vi "KB-产品统计.vi"(7 "file path (dialog if empty)":path=path "E:/Users/HEZHIFENG/Desktop/image Picture#2 Balck/20160927.xls", 9 "限位表格":string[][](table)=[["0.2", "0", "0.25", "0", "0.1", "0", "10", "-10", "金色"], ["0.2", "0", "0.25", "0", "0.1", "0", "10", "-10", "金色"], ["0.2", "0", "0.25", "0", "0.1", "0", "10", "-10", "金色"], ["0.2", "0", "0.25", "0", "0.1", "0", "10", "-10", "金色"], ["0.2", "0", "0.25", "0", "0.1", "0", "10", "-10", "金色"], ["0.2", "0", "0.25", "0", "0.1", "0", "10", "-10", "金色"], ["0.2", "0", "0.25", "0", "0.1", "0", "10", "-10", "银色"], ["0.2", "0", "0.25", "0", "0.1", "0", "10", "-10", "银色"], ["0.2", "0", "0.25", "0", "0.1", "0", "10", "-10", "银色"], ["0.2", "0", "0.25", "0", "0.1", "0", "10", "-10", "银色"], ["0.2", "0", "0.25", "0", "0.1", "0", "10", "-10", "金色"], ["0.2", "0", "0.25", "0", "0.1", "0", "10", "-10", "金色"], ["0.2", "0", "0.25", "0", "0.1", "0", "10", "-10", "金色"], ["0.2", "0", "0.25", "0", "0.1", "0", "10", "-10", "金色"], ["0.2", "0", "0.25", "0", "0.1", "0", "10", "-10", "金色"], ["0.2", "0", "0.25", "0", "0.1", "0", "10", "-10", "金色"], ["0.2", "0", "0.25", "0", "0.1", "0", "10", "-10", "金色"], ["0.2", "0", "0.25", "0", "0.1", "0", "10", "-10", "金色"], ["0.2", "0", "0.25", "0", "0.1", "0", "10", "-10", "金色"], ["0.2", "0", "0.25", "0", "0.1", "0", "10", "-10", "金色"], ["0.2", "0", "0.25", "0", "0.1", "0", "10", "-10", "金色"], ["0.2", "0", "0.25", "0", "0.1", "0", "10", "-10", "金色"], ["0.2", "0", "0.25", "0", "0.1", "0", "10", "-10", "金色"], ["0.2", "0", "0.25", "0", "0.1", "0", "10", "-10", "金色"], ["0.2", "0", "0.25", "0", "0.1", "0", "10", "-10", "金色"], ["0.2", "0", "0.25", "0", "0.1", "0", "10", "-10", "金色"], ["0.2", "0", "0.25", "0", "0.1", "0", "10", "-10", "金色"], ["0.2", "0", "0.25", "0", "0.1", "0", "10", "-10", "金色"], ["0.2", "0", "0.25", "0", "0.1", "0", "10", "-10", "金色"], ["0.2", "0", "0.25", "0", "0.1", "0", "10", "-10", "金色"], ["0.2", "0", "0.25", "0", "0.1", "0", "10", "-10", "金色"]], 10 "结束时间":string(combo)="24", 11 "起始时间":string(combo)="01") -> (1 "Tab同心度":string[][](table)=[["0", "0", "0", "0", "0"]], 2 "Tab高度差":string[][](table)=[["165", "20", "1", "0", "0"]], 3 "Tab":string[][](table)=[["1", "", "255", "N/A", "N/A", "N/A", "465"], ["2", "", "N/A", "250", "N/A", "N/A", "N/A"], ["3", "", "N/A", "N/A", "20", "N/A", "N/A"], ["4", "", "N/A", "N/A", "N/A", "10", "N/A"]])   [LabVIEW 2015]
uses:
  <vilib>/Utility/miscctls.llb/LVRowAndColumnTypeDef.ctl
  <vilib>/Utility/file.llb/Read Delimited Spreadsheet (string).vi
panel:
  out "数组":string[](array[string])
  out "子数组":string[](array[string])
  out "已删除元素的数组子集":string[][](array[string])
  out "输出簇":T1
  out "OK 个数":string
  out "混装 个数":string
  out "同心度NG 个数":string
  out "高度差NG 个数":string
  out "漏料个数":string
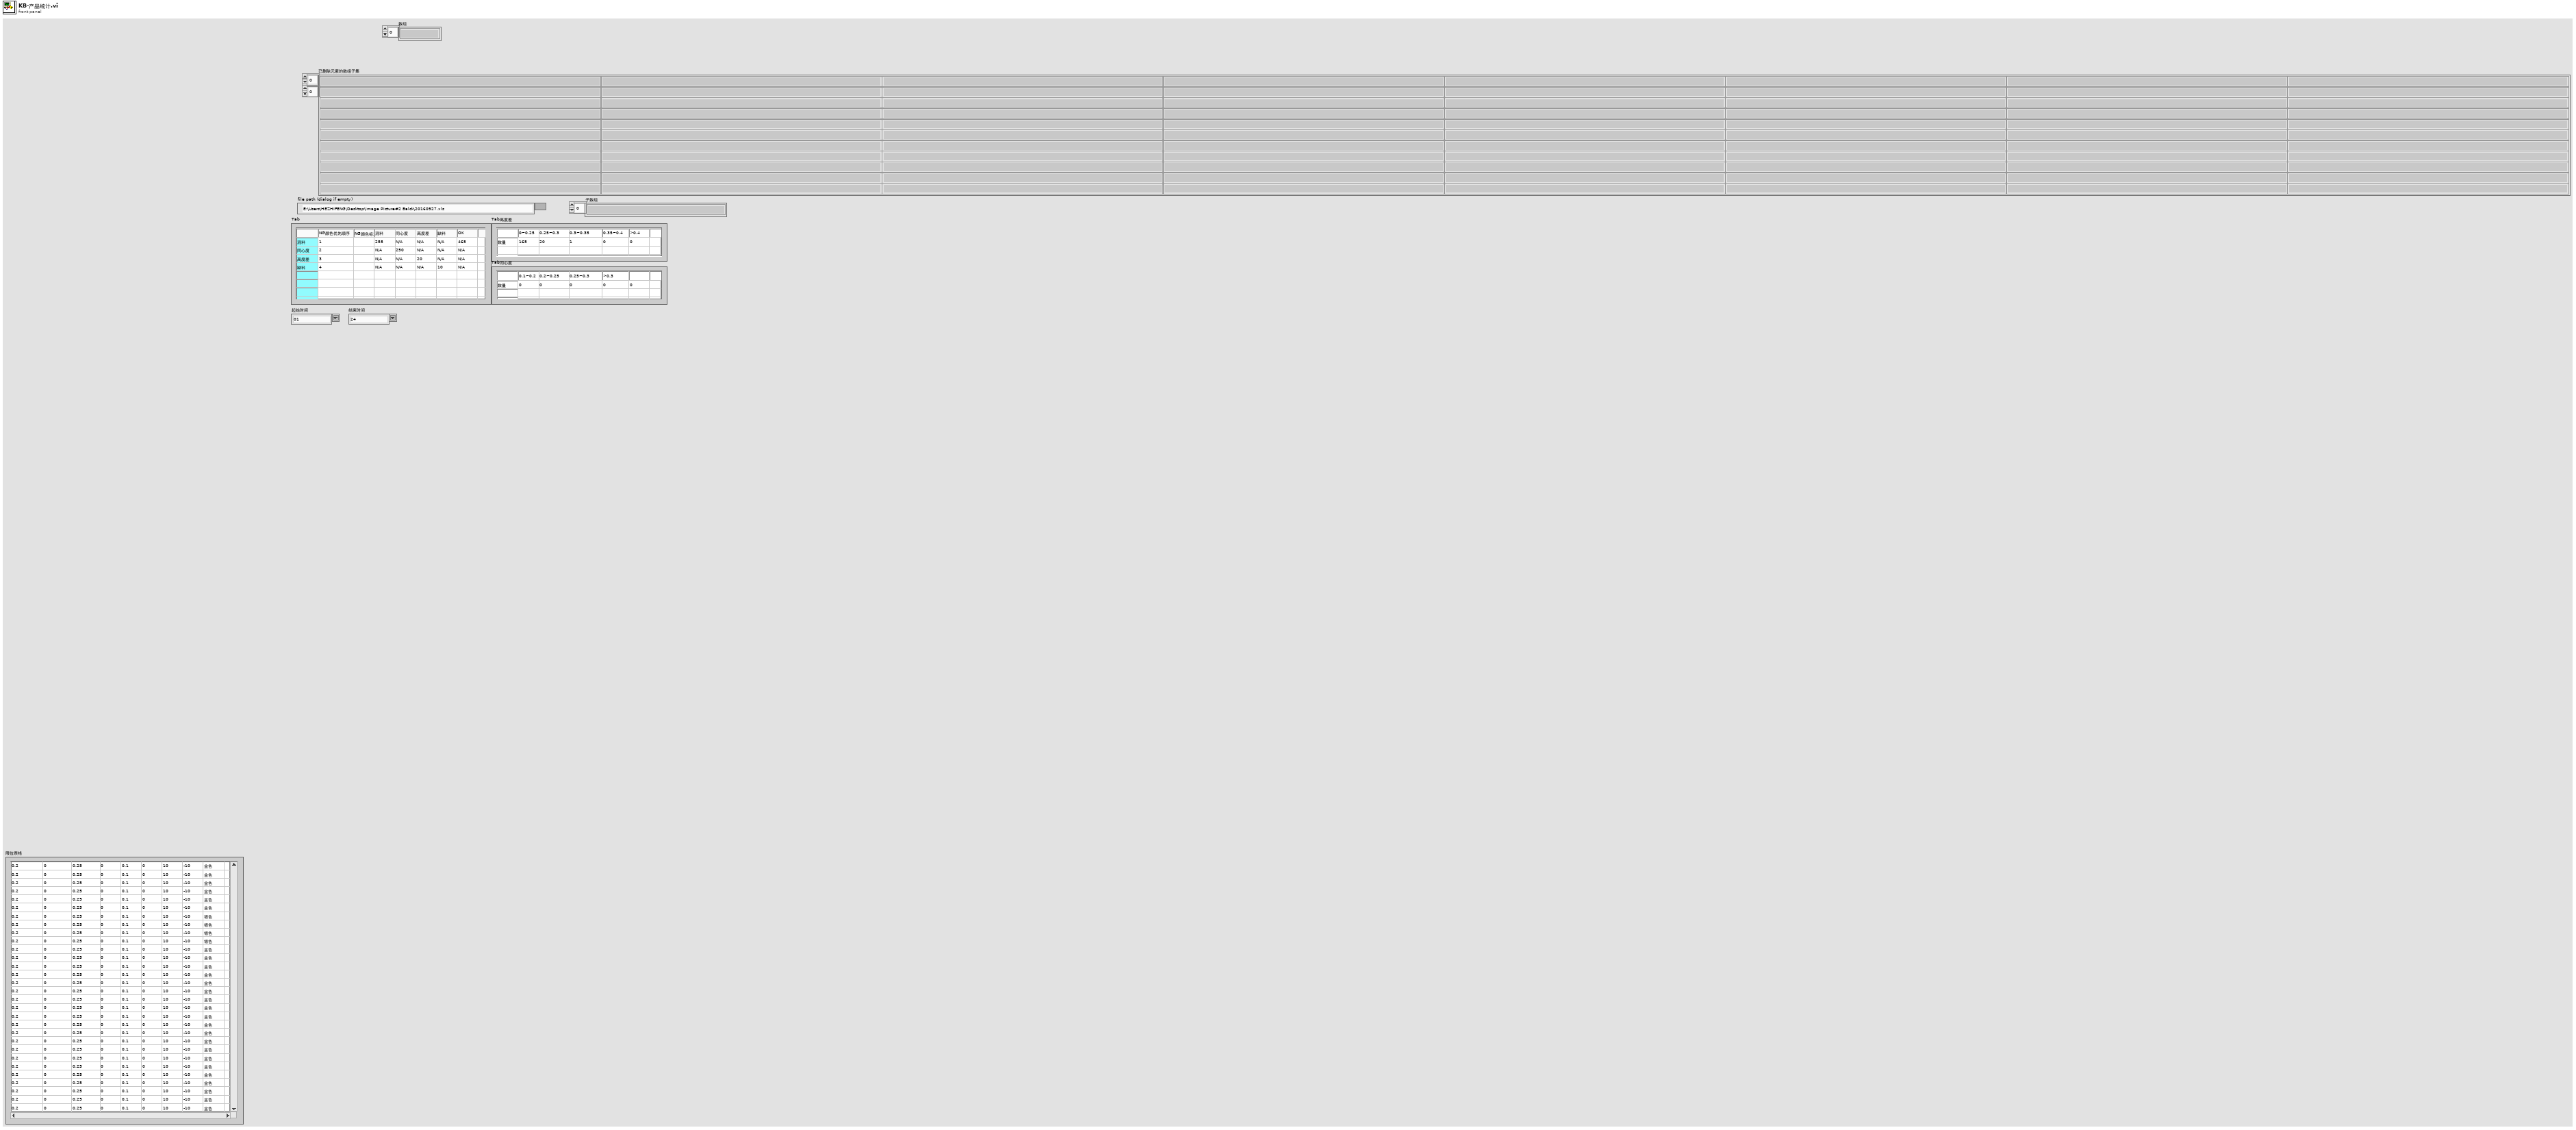
[diagram p1: front panel]
types:
  T1 = cluster{"漏料个数 ":string, "高度差NG 个数":string, "同心度NG 个数 ":string, "混装 个数 ":string, "OK 个数":string}
  T2 = typedef "LVRowAndColumnTypeDef.ctl" = cluster{"Row":i32, "Column":i32}
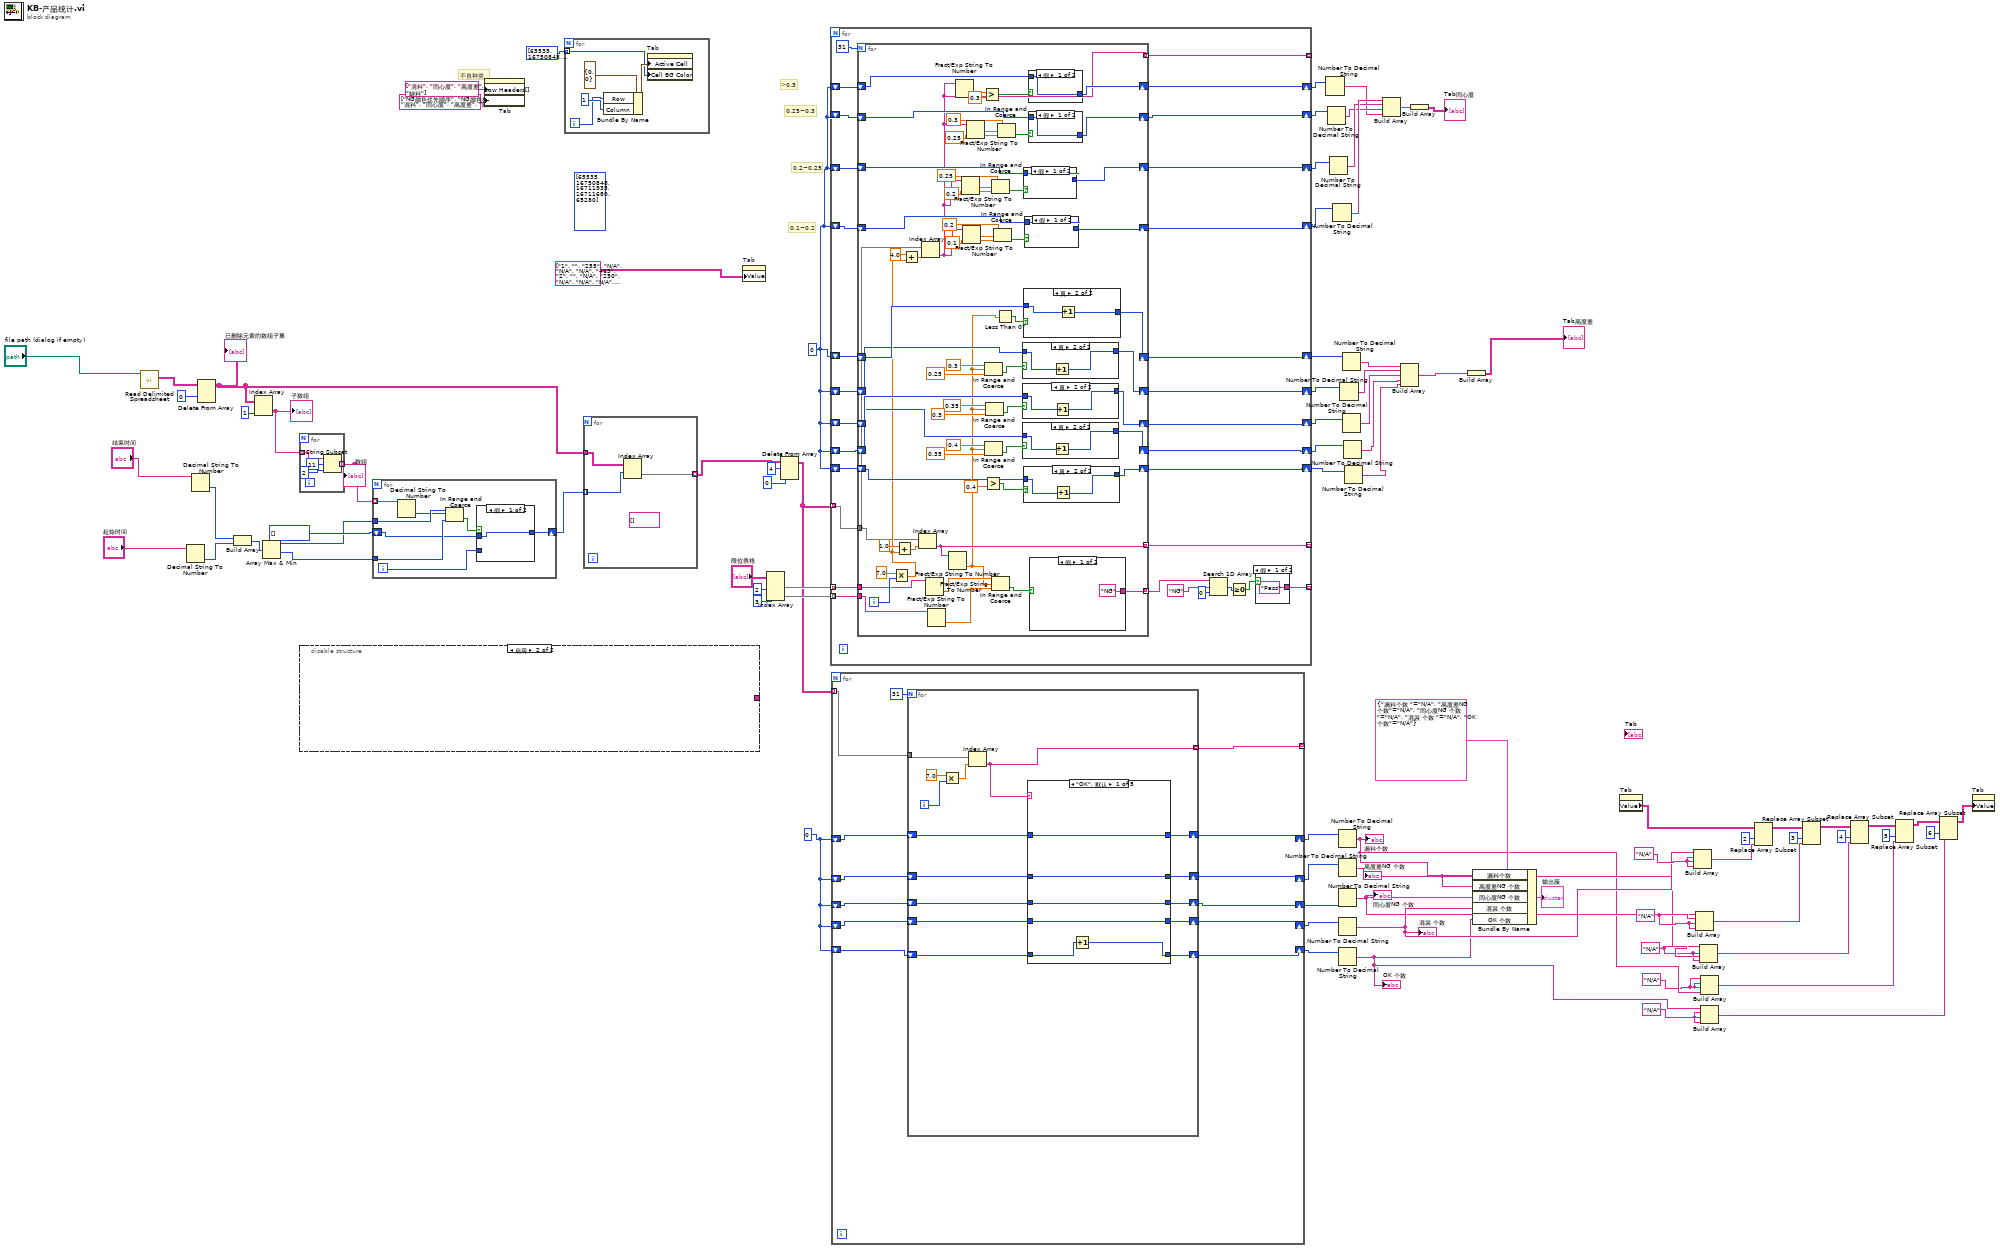
[diagram p0: block diagram]
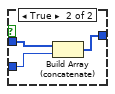
[diagram p2: hidden frame]
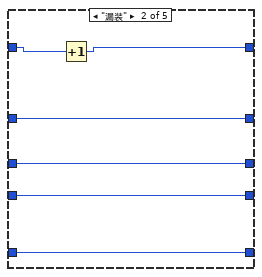
[diagram p3: hidden frame]
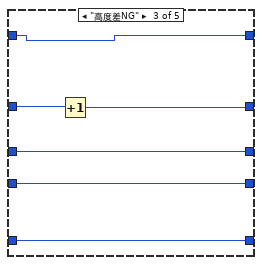
[diagram p4: hidden frame]
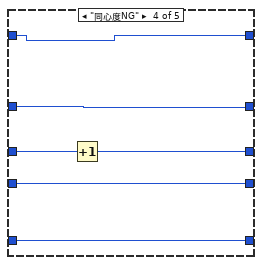
[diagram p5: hidden frame]
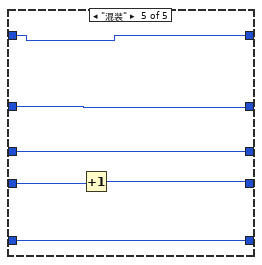
[diagram p6: hidden frame]
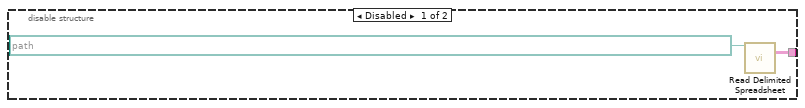
[diagram p7: hidden frame]
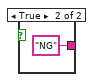
[diagram p8: hidden frame]
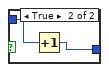
[diagram p9: hidden frame]
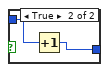
[diagram p10: hidden frame]
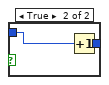
[diagram p11: hidden frame]
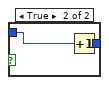
[diagram p12: hidden frame]
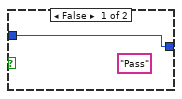
[diagram p17: hidden frame]
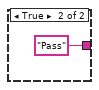
[diagram p18: hidden frame]
diagram:
  w26 = 0 ("禁用的索引 (列)")
  w60 = "N/A" ("元素")
  w39 = "N/A" ("元素")
  w41 = "N/A" ("元素")
  w43 = "N/A" ("元素")
  w62 = "N/A" ("元素")
  w70 = 0
  (unwired) u32[] [65535, 16750848, 16711935, 16711680, 65280]
  # ">0.3"
  # "0.25~0.3"
  # "0.2~0.25"
  # "0.1~0.2"
  # "不良种类"
  n1 = call-poly <vilib>:"Read Delimited Spreadsheet.vi"("file path (dialog if empty)"="file path (dialog if empty)") -> ("all rows"=w81:string[][])  [unwired: 9 in, 5 out]
  n2 = Decimal String To Number(string="起始时间") -> (number=w3:i32)  [unwired: 2 in, 1 out]
  n3 = Decimal String To Number(string="结束时间") -> (number=w5:i32)  [unwired: 2 in, 1 out]
  n4 = Delete From Array(array=w81, index (row)=0 ("索引 (行)")) -> (array with subset deleted=w9:string[][])  [unwired: 2 in, 1 out]
  "已删除元素的数组子集" <- w9
  n5 = Build Array(w5, w3) -> (w4:i32[])
  n6 = Index Array(array=w9, index (col)=1 ("禁用的索引 (列)")) -> (element=w14:string[])  [unwired: 1 in]
  "子数组" <- w14
  n7 = Array Max & Min(array=w4) -> (max value=w1:i32, min value=w2:i32)  [unwired: 2 out]
  n8 = for {
    tunnel: w14 -> [w90] mode=indexing
    tunnel: [w87] -> w13 mode=indexing
    n9 = String Subset(string=w90, offset (0)=11 ("偏移量(0)"), length (rest)=2 ("长度（剩余）")) -> (substring=w87:string)
  }
  "数组" <- w13
  n10 = disable-structure shown="启用" {
    disable-tunnel: [w91 _] -> _
    frame Disabled {
      n11 = call-poly <vilib>:"Read Delimited Spreadsheet.vi"("file path (dialog if empty)"=path "G:/项目/KN-Software/#1/KNight Back Housing/Source Code/Template Program/potteryTemplete/ALL Tolerance Param.txt") -> ("all rows"=w91:string[][])  [unwired: 9 in, 5 out]
    }
    frame Enabled {
    }
  }
  n12 = for {
    tunnel: w13 -> [w100] mode=indexing
    tunnel: w1 -> [w99]
    tunnel: w2 -> [w98]
    shift-right: [w93] -> w8
    shift-left: i32[] [] -> [w94]
    i -> [w96]
    n13 = Decimal String To Number(string=w100) -> (number=w97:i32)  [unwired: 2 in, 1 out]
    n14 = In Range and Coerce(upper limit=w99, x=w97, lower limit=w98) -> (In Range?=w95:bool)  [unwired: 1 out]
    n15 = case shown="假" w95 {
      tunnel: w96 -> [_ w102]
      tunnel: w94 -> [w101 w104]
      tunnel: [w101 w103] -> w93
      frame False {
      }
      frame True {
        n16 = Build Array (concatenate)(w104, w102) -> (w103:i32[])
      }
    }
  }
  n17 = property on="Tab" class="Tbl (严格)"("Row Headers[]"=string[] ["混料", "同心度", "高度差", "缺料"] ("行首字符串[]"), "Column Headers[]"=string[] ["NG颜色优先顺序", "NG颜色标示", "混料", "同心度", "高度差", "缺料", "OK"] ("列首字符串[]")) -> ()  [unwired: 2 in, 2 out]
  n18 = for {
    tunnel: u32[] [65535, 16750848, 16711935, 16711680] -> [w105] mode=indexing
    i -> [w106]
    n19 = Bundle By Name(cluster=T2 {"Row"=0, "Column"=0} ("活动单元格:活动单元格"), "Row"=w106, "Column"=1 ("Row")) -> (w108:T2)
    n20 = property on="Tab" class="Tbl (严格)"("Active Cell"=w108, "Cell BG Color"=w105) -> ()  [unwired: 2 in, 2 out]
  }
  n21 = for {
    tunnel: w9 -> [w112]
    tunnel: w8 -> [w111] mode=indexing
    tunnel: [w110] -> w7 mode=indexing
    (unwired) string[] []
    n22 = Index Array(array=w112, index (row)=w111) -> (element=w110:string[])  [unwired: 1 in]
  }
  n23 = property on="Tab" class="Tbl (严格)"("Value"=string[][] [["1", "", "255", "N/A", "N/A", "N/A", "465"], ["2", "", "N/A", "250", "N/A", "N/A", "N/A"], ["3", "", "N/A", "N/A", "20", "N/A", "N/A"], ["4", "", "N/A", "N/A", "N/A", "10", "N/A"]]) -> ()  [unwired: 2 in, 2 out]
  n24 = Index Array(array="限位表格", index (col) #1=2 ("禁用的索引 (列)"), index (col) #2=3 ("索引 (列)")) -> (element #1=w73:string[], element #2=w72:string[])  [unwired: 2 in]
  n25 = Delete From Array(array=w7, length=4 ("长度"), index (col)=0 ("禁用的索引 (列)")) -> (array with subset deleted=w71:string[][])  [unwired: 1 in, 1 out]
  n26 = for {
    tunnel: w71 -> [w142] mode=indexing
    tunnel: [w140] -> _ mode=indexing
    tunnel: w73 -> [w139] mode=indexing
    tunnel: w72 -> [w138] mode=indexing
    tunnel: [w132] -> _ mode=indexing
    shift-right: [w130] -> w38
    shift-left: w26 -> [w131]
    shift-right: [w128] -> w37
    shift-left: w26 -> [w129]
    shift-right: [w126] -> w36
    shift-left: w26 -> [w127]
    shift-right: [w124] -> w35
    shift-left: w26 -> [w125]
    shift-right: [w122] -> w34
    shift-left: w26 -> [w123]
    shift-right: [w120] -> w22
    shift-left: w26 -> [w121]
    shift-right: [w118] -> w23
    shift-left: w26 -> [w119]
    shift-right: [w116] -> w24
    shift-left: w26 -> [w117]
    shift-right: [w114] -> w25
    shift-left: w26 -> [w115]
    tunnel: [w113] -> _ mode=indexing
    n27 = for {
      N: 31 -> [_]
      tunnel: w142 -> [w146]
      tunnel: [w200] -> w140 mode=indexing
      tunnel: w139 -> [w204]
      tunnel: w138 -> [w202]
      tunnel: [w198] -> w137 mode=indexing
      shift-right: [w194] -> w130
      shift-left: w131 -> [w195]
      shift-right: [w189] -> w128
      shift-left: w129 -> [w190]
      shift-right: [w184] -> w126
      shift-left: w127 -> [w185]
      shift-right: [w179] -> w124
      shift-left: w125 -> [w180]
      shift-right: [w175] -> w122
      shift-left: w123 -> [w176]
      shift-right: [w164] -> w120
      shift-left: w121 -> [w165]
      shift-right: [w158] -> w118
      shift-left: w119 -> [w159]
      shift-right: [w152] -> w116
      shift-left: w117 -> [w153]
      shift-right: [w147] -> w114
      shift-left: w115 -> [w148]
      tunnel: [w145] -> w113 mode=indexing
      i -> [w205]
      n28 = Multiply(x=7.0, y=w205) -> (x*y=w170:dbl)
      n29 = Add(x=1.0, y=w170) -> (x+y=w196:dbl)
      n30 = Add(x=4.0, y=w170) -> (x+y=w172:dbl)
      n31 = Index Array(array=w146, index=w196) -> (element=w200:string)
      n32 = Index Array(array=w146, index=w172) -> (element=w145:string)
      n33 = Fract/Exp String To Number(string=w204) -> (number=w203:dbl)  [unwired: 3 in, 1 out]
      n34 = Fract/Exp String To Number(string=w202) -> (number=w201:dbl)  [unwired: 3 in, 1 out]
      n35 = Fract/Exp String To Number(string=w200) -> (number=w174:dbl)  [unwired: 3 in, 1 out]
      n36 = Fract/Exp String To Number(string=w145) -> (number=w151:dbl)  [unwired: 3 in, 1 out]
      n37 = Fract/Exp String To Number(string=w145) -> (number=w160:dbl)  [unwired: 3 in, 1 out]
      n38 = Fract/Exp String To Number(string=w145) -> (number=w169:dbl)  [unwired: 3 in, 1 out]
      n39 = Fract/Exp String To Number(string=w145) -> (number=w157:dbl)  [unwired: 3 in, 1 out]
      n40 = Greater?(x=w151, y=0.3) -> (0:w149:bool)
      n41 = Greater?(x=w174, y=0.4) -> (0:w177:bool)
      n42 = In Range and Coerce(upper limit=0.3 ("上限"), x=w174, lower limit=0.25 ("下限")) -> (In Range?=w193:bool)  [unwired: 1 out]
      n43 = In Range and Coerce(upper limit=0.4 ("上限"), x=w174, lower limit=0.35 ("下限")) -> (In Range?=w183:bool)  [unwired: 1 out]
      n44 = In Range and Coerce(upper limit=0.35 ("上限"), x=w174, lower limit=0.3 ("下限")) -> (In Range?=w186:bool)  [unwired: 1 out]
      n45 = In Range and Coerce(upper limit=0.25 ("上限"), x=w160, lower limit=0.2 ("下限")) -> (In Range?=w163:bool)  [unwired: 1 out]
      n46 = In Range and Coerce(upper limit=w203, x=w174, lower limit=w201) -> (In Range?=w199:bool)  [unwired: 1 out]
      n47 = In Range and Coerce(upper limit=0.2 ("上限"), x=w169, lower limit=0.1 ("下限")) -> (In Range?=w166:bool)  [unwired: 1 out]
      n48 = Less Than 0?(x=w174) -> (x < 0?=w173:bool)
      n49 = In Range and Coerce(upper limit=0.3 ("上限"), x=w157, lower limit=0.25 ("下限")) -> (In Range?=w154:bool)  [unwired: 1 out]
      n50 = case shown="真" w193 {
        tunnel: w190 -> [w228 w230]
        tunnel: [w228 w229] -> w189
        frame False {
        }
        frame True {
          n51 = Increment(x=w230) -> (x+1=w229:i32)
        }
      }
      n52 = case shown="真" w183 {
        tunnel: [w222 w224] -> w179
        tunnel: w180 -> [w222 w223]
        frame False {
        }
        frame True {
          n53 = Increment(x=w223) -> (x+1=w224:i32)
        }
      }
      n54 = case shown="真" w186 {
        tunnel: [w225 w227] -> w184
        tunnel: w185 -> [w225 w226]
        frame False {
        }
        frame True {
          n55 = Increment(x=w226) -> (x+1=w227:i32)
        }
      }
      n56 = case shown="假" w163 {
        tunnel: w159 -> [w213 w215]
        tunnel: [w213 w214] -> w158
        frame False {
        }
        frame True {
          n57 = Increment(x=w215) -> (x+1=w214:i32)
        }
      }
      n58 = case shown="真" w177 {
        tunnel: [w219 w221] -> w175
        tunnel: w176 -> [w219 w220]
        frame False {
        }
        frame True {
          n59 = Increment(x=w220) -> (x+1=w221:i32)
        }
      }
      n60 = case shown="真" w173 {
        tunnel: w195 -> [w231 w233]
        tunnel: [w231 w232] -> w194
        frame False {
          (unwired) "Pass"
        }
        frame True {
          n61 = Increment(x=w233) -> (x+1=w232:i32)
        }
      }
      n62 = case shown="假" w166 {
        tunnel: w165 -> [w216 w218]
        tunnel: [w216 w217] -> w164
        frame False {
        }
        frame True {
          n63 = Increment(x=w218) -> (x+1=w217:i32)
        }
      }
      n64 = case shown="假" w149 {
        tunnel: w148 -> [w207 w209]
        tunnel: [w207 w208] -> w147
        frame False {
        }
        frame True {
          n65 = Increment(x=w209) -> (x+1=w208:i32)
        }
      }
      n66 = case shown="假" w154 {
        tunnel: w153 -> [w210 w212]
        tunnel: [w210 w211] -> w152
        frame False {
        }
        frame True {
          n67 = Increment(x=w212) -> (x+1=w211:i32)
        }
      }
      n68 = case shown="假" w199 {
        tunnel: ["NG" "Pass"] -> w198
        frame False {
        }
        frame True {
        }
      }
    }
    n69 = Search 1D Array(1D array=w137, element="NG" ("元素"), start index (0)=0 ("开始索引(0)")) -> (index of element=w134:i32)
    n70 = Greater Or Equal To 0?(x=w134) -> (x >= 0?=w133:bool)
    n71 = case shown="假" w133 {
      tunnel: ["Pass" ("元素") "NG" ("元素")] -> w132
      frame False {
      }
      frame True {
      }
    }
  }
  n72 = for {
    tunnel: w71 -> [w247] mode=indexing
    tunnel: [w246] -> _ mode=indexing
    shift-right: [w241] -> w69
    shift-left: w70 -> [w245]
    shift-right: [w240] -> w68
    shift-left: w70 -> [w244]
    shift-right: [w239] -> w67
    shift-left: w70 -> [w243]
    shift-right: [w238] -> w66
    shift-left: w70 -> [w242]
    shift-right: [w236] -> w65
    shift-left: w70 -> [w237]
    n73 = for {
      N: 31 -> [_]
      tunnel: w247 -> [w262]
      tunnel: [w259] -> w246 mode=indexing
      shift-right: [w257] -> w241
      shift-left: w245 -> [w258]
      shift-right: [w255] -> w240
      shift-left: w244 -> [w256]
      shift-right: [w253] -> w239
      shift-left: w243 -> [w254]
      shift-right: [w251] -> w238
      shift-left: w242 -> [w252]
      shift-right: [w249] -> w236
      shift-left: w237 -> [w250]
      i -> [w260]
      n74 = Multiply(x=7.0, y=w260) -> (x*y=w261:dbl)
      n75 = Index Array(array=w262, index=w261) -> (element=w259:string)
      n76 = case shown="\"OK\", 默认" w259 {
        tunnel: w258 -> [w269 w275 w279 w286 w293]
        tunnel: [w269 w274 w279 w286 w293] -> w257
        tunnel: w256 -> [w268 w273 w278 w285 w292]
        tunnel: [w268 w273 w277 w285 w292] -> w255
        tunnel: w254 -> [w267 w272 w281 w284 w291]
        tunnel: [w267 w272 w281 w283 w291] -> w253
        tunnel: w252 -> [w266 w271 w280 w287 w290]
        tunnel: [w266 w271 w280 w287 w289] -> w251
        tunnel: w250 -> [w265 w270 w276 w282 w288]
        tunnel: [w264 w270 w276 w282 w288] -> w249
        frame "OK", Default {
          n77 = Increment(x=w265) -> (x+1=w264:i32)
        }
        frame "漏装" {
          n78 = Increment(x=w275) -> (x+1=w274:i32)
        }
        frame "高度差NG" {
          n79 = Increment(x=w278) -> (x+1=w277:i32)
        }
        frame "同心度NG" {
          n80 = Increment(x=w284) -> (x+1=w283:i32)
        }
        frame "混装" {
          n81 = Increment(x=w290) -> (x+1=w289:i32)
        }
      }
    }
  }
  n82 = Number To Decimal String(number=w25) -> (decimal integer string=w16:string)  [unwired: 1 in]
  n83 = Number To Decimal String(number=w24) -> (decimal integer string=w17:string)  [unwired: 1 in]
  n84 = Number To Decimal String(number=w23) -> (decimal integer string=w18:string)  [unwired: 1 in]
  n85 = Number To Decimal String(number=w22) -> (decimal integer string=w19:string)  [unwired: 1 in]
  n86 = Number To Decimal String(number=w69) -> (decimal integer string=w40:string)  [unwired: 1 in]
  "漏料个数" <- w40
  n87 = Number To Decimal String(number=w68) -> (decimal integer string=w42:string)  [unwired: 1 in]
  "高度差NG 个数" <- w42
  n88 = Number To Decimal String(number=w67) -> (decimal integer string=w44:string)  [unwired: 1 in]
  "同心度NG 个数" <- w44
  n89 = Number To Decimal String(number=w66) -> (decimal integer string=w61:string)  [unwired: 1 in]
  "混装 个数" <- w61
  n90 = Number To Decimal String(number=w65) -> (decimal integer string=w59:string)  [unwired: 1 in]
  "OK 个数" <- w59
  n91 = Number To Decimal String(number=w37) -> (decimal integer string=w32:string)  [unwired: 1 in]
  n92 = Number To Decimal String(number=w38) -> (decimal integer string=w33:string)  [unwired: 1 in]
  n93 = Number To Decimal String(number=w36) -> (decimal integer string=w31:string)  [unwired: 1 in]
  n94 = Number To Decimal String(number=w35) -> (decimal integer string=w30:string)  [unwired: 1 in]
  n95 = Number To Decimal String(number=w34) -> (decimal integer string=w29:string)  [unwired: 1 in]
  n96 = Build Array(w19, w18, w17, w16) -> (w21:string[])
  n97 = Build Array(w33, w32, w31, w30, w29) -> (w28:string[])
  n98 = Build Array(w21) -> (→"Tab同心度":string[][])
  n99 = Build Array(w28) -> (→"Tab高度差":string[][])
  n100 = Bundle By Name(cluster=T1 {"漏料个数 "="N/A", "高度差NG 个数"="N/A", "同心度NG 个数 "="N/A", "混装 个数 "="N/A", "OK 个数"="N/A"}, "漏料个数"=w40, "高度差NG 个数"=w42, "同心度NG 个数"=w44, "混装 个数"=w61, "OK 个数"=w59) -> (→"输出簇":T1)
  n101 = property on="Tab" class="Tbl (严格)"() -> ("Value"=w6:string[][])  [unwired: 2 in, 2 out]
  n102 = Build Array(w61, w62, w62, w62) -> (w49:string[])
  n103 = Build Array(w43, w44, w43, w43) -> (w48:string[])
  n104 = Build Array(w41, w41, w42, w41) -> (w47:string[])
  n105 = Build Array(w39, w39, w39, w40) -> (w46:string[])
  n106 = Build Array(w59, w60, w60, w60) -> (w45:string[])
  n107 = Replace Array Subset(array=w6, new element=w49, index (col)=2 ("禁用的索引 (列)")) -> (w54:string[][])  [unwired: 1 in]
  n108 = Replace Array Subset(array=w54, new element=w48, index (col)=3 ("禁用的索引 (列)")) -> (w53:string[][])  [unwired: 1 in]
  n109 = Replace Array Subset(array=w53, new element=w47, index (col)=4 ("禁用的索引 (列)")) -> (w52:string[][])  [unwired: 1 in]
  n110 = Replace Array Subset(array=w52, new element=w46, index (col)=5 ("禁用的索引 (列)")) -> (w51:string[][])  [unwired: 1 in]
  n111 = Replace Array Subset(array=w51, new element=w45, index (col)=6 ("禁用的索引 (列)")) -> (w50:string[][])  [unwired: 1 in]
  n112 = property on="Tab" class="Tbl (严格)"("Value"=w50) -> ()  [unwired: 2 in, 2 out]
